vi "Configure Hardware.vi"(8 "error in (no error)":errorcluster, 10 "Calibration Task in":refnum<k21>, 11 "Acq Settings in":T1 {"Config Settings"."Simulated Sensor Injection" scale=0.0..100.0}) -> (0 "error out":errorcluster, 2 "Calibration Task out":refnum<k21>, 3 "Acq Settings out":T1 {"Config Settings"."Simulated Sensor Injection" scale=0.0..100.0})   [LabVIEW 2026, in "Acquisition.lvlib"]
doc: "Configure the hardware."
uses:
  Acquisition.lvlib
  controls/UI/Acq Settings.ctl
  Instrument Specifications Configuration.ctl
  Instrument Specifications Cluster Configuration.ctl
  controls/UI/Measurement Role.ctl
  controls/UI/Config Settings.ctl
  <vilib>/DAQmx/configure/timing.llb/DAQmx Timing (Sample Clock).vi
  Settings/Settings.lvlib
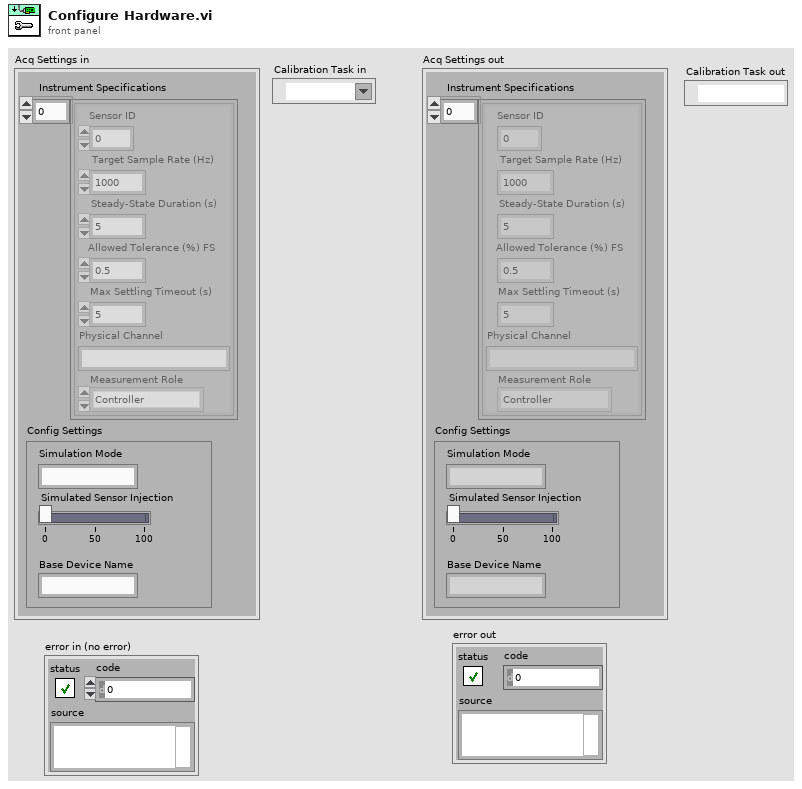
[diagram p1: front panel]
types:
  T1 = typedef "Acq Settings.ctl" = cluster{"Instrument Specifications":T2, "Config Settings":T5}
  T2 = typedef "Acquisition.lvlib/Instrument Specifications Configuration.ctl" = T3[]
  T3 = typedef "Acquisition.lvlib/Instrument Specifications Cluster Configuration.ctl" = cluster{"Sensor ID":i32, "Target Sample Rate (Hz)":dbl, "Steady-State Duration (s)":i32, "Allowed Tolerance (%) FS":dbl, "Max Settling Timeout (s)":i32, "Physical Channel":string, "Measurement Role":T4}
  T4 = typedef "Settings.lvlib/Measurement Role.ctl" = enum16{"Controller", "Reference", "UUT", "Disable", "All"}
  T5 = typedef "Config Settings.ctl" = cluster{"Simulated Sensor Injection":dbl, "Base Device Name":string, "Simulation Mode":string}
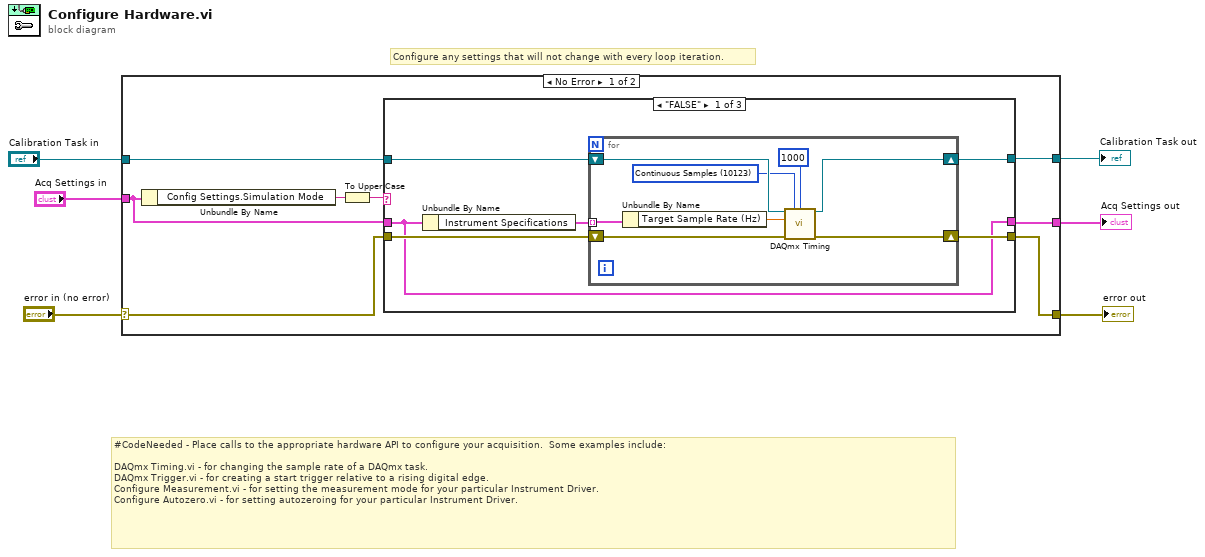
[diagram p0: block diagram]
diagram:
  # "Configure any settings that will not change with every loop iteration."
  # "#CodeNeeded - Place calls to the appropriate hardware API to configure your acquisition.  Some examples include:\n\nDAQmx Timing.vi - for changing the sample rate of a DAQmx task.\nDAQmx Trigger.vi - for creating a start trigger relative to a rising digital edge.\nConfigure Measurement.vi - for setting the measurement mode for your particular Instrument Driver.\nConfigure Autozero.vi - for setting autozeroing for your particular Instrument Driver."
  n1 = case shown="No Error" "error in (no error)" {
    selector: "error in (no error)" -> [w13 w37]
    tunnel: [w12 w37] -> w5
    tunnel: "Acq Settings in" -> [w7 w36]
    tunnel: [w10 w36] -> w3
    tunnel: "Calibration Task in" -> [w14 w35]
    tunnel: [w11 w35] -> w1
    frame No Error {
      n2 = Unbundle By Name(w7) -> ("Config Settings.Simulation Mode"=w9:string)
      n3 = To Upper Case(1:w9) -> (0:w8:string)
      n4 = case shown="\"FALSE\"" w8 {
        tunnel: w14 -> [w20 w29 w34]
        tunnel: w13 -> [w18 w31 w32]
        tunnel: [w17 w31 w32] -> w12
        tunnel: [w19 w29 w34] -> w11
        tunnel: [w15 w30 w33] -> w10
        tunnel: w7 -> [w15 w30 w33]
        frame "FALSE" {
          n5 = Unbundle By Name(w15) -> ("Instrument Specifications"=w16:T2)
          n6 = for {
            shift-right: [w25] -> w19
            shift-left: w20 -> [w28]
            shift-right: [w23] -> w17
            shift-left: w18 -> [w24]
            tunnel: w16 -> [w22] mode=indexing
            w27 = 10123 items=["Finite Samples"=10178, "Continuous Samples"=10123, "Hardware Timed Single Point"=12522] ("sample mode")
            n7 = Unbundle By Name(w22) -> ("Target Sample Rate (Hz)"=w21:dbl)
            n8 = call-poly <vilib>:"DAQmx Timing.vi"("task/channels in"=w28, "sample mode"=w27, "samples per channel"=1000, "rate"=w21, "error in"=w24) -> ("task out"=w25:refnum<k21>, "error out"=w23:errorcluster)  [unwired: 9 in]
          }
        }
        frame "TRUE" {
        }
        frame Default {
        }
      }
    }
    frame Error {
    }
  }
  "error out" <- w5
  "Acq Settings out" <- w3
  "Calibration Task out" <- w1
